vi "PH_Switch.set Default.vi"(0 "i ref in":refnum<vi>, 5 "error in":errorcluster) -> (14 "i ref out":refnum<vi>, 19 "error out":errorcluster)   [LabVIEW 2014, in "PH_Switch.lvlib"]
doc: "This VI sets the default value."
uses:
  PH_Switch.lvlib
  CS_Core/CSSystem/CSSystemLib/CSSystemLib.lvlib
  CS_Core/BaseProcess/BaseProcess.lvlib
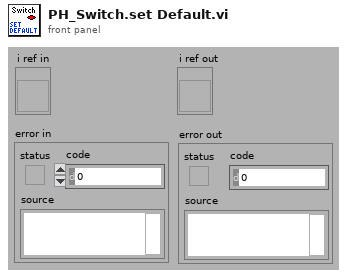
[diagram p1: front panel]
types:
  T1 = typedef "BaseProcess.lvlib/BaseProcess.i attribute.ctl" = cluster{"EventStatus":string, "EventError":i32, "PresetEvtWatchD":i32, "PresetPdcWatchD":i32, "EventTimeout":i32, "PeriodicInterval":i32, "Interface":string[], "Address":string[], "Special":string[], "PeriodicError":i32, "PeriodicStatus":string, "SuperProc":string, "Descriptors":T2[], "CaseRef":refnum<vi>, "PdcRef":refnum<vi>, "Thread Ref":refnum<vi>, "eventErrorID":i32, "eventStatusID":i32, "periodicErrorID":i32, "periodicStatusID":i32, "pdcCtrID":i32}
  T2 = typedef "BaseProcess.lvlib/BaseProcess.descriptor definition.ctl" = cluster{"selector":string, "descriptor":T3}
  T3 = typedef "BaseProcess.lvlib/BaseProcess.descriptor string definition.ctl" = string
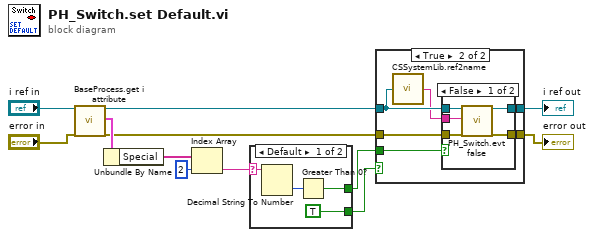
[diagram p0: block diagram]
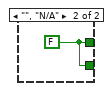
[diagram p2: hidden frame]
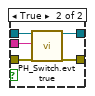
[diagram p4: hidden frame]
diagram:
  n1 = call "BaseProcess.get i attribute.vi"("i ref in"="i ref in", "error in (no error)"="error in") -> ("i ref out"=w2:refnum<vi>, "i attribute"=w10:T1, "error out"=w1:errorcluster)  [unwired: 15 in]
  n2 = Unbundle By Name(w10) -> ("Special"=w9:string[])
  n3 = Index Array(array=w9, index=2) -> (element=w7:string)
  n4 = case shown="Default" w7 {
    selector: w7 -> [w15 _]
    tunnel: [TRUE w17] -> w6
    tunnel: [w13 w17] -> w5
    frame Default {
      n5 = Decimal String To Number(string=w15) -> (number=w14:i32)  [unwired: 2 in, 1 out]
      n6 = Greater Than 0?(x=w14) -> (x > 0?=w13:bool)
    }
    frame "", "N/A" {
      w17 = FALSE
    }
  }
  n7 = case shown="True" w6 {
    tunnel: [w19 w25] -> w11
    tunnel: w1 -> [w18 w24]
    tunnel: [w18 w23] -> w12
    tunnel: w5 -> [_ w22]
    tunnel: w2 -> [w19 w21]
    frame False {
    }
    frame True {
      n8 = call "CSSystemLib.ref2name.vi"("obj refnum"=w21) -> ("name"=w20:string)
      n9 = case shown="False" w22 {
        tunnel: w21 -> [w30 w35]
        tunnel: [w29 w34] -> w25
        tunnel: w24 -> [w28 w33]
        tunnel: [w27 w32] -> w23
        tunnel: w20 -> [w26 w31]
        frame False {
          n10 = call "PH_Switch.evt false.vi"("i ref in"=w30, "Instance"=w26, "error in (no error)"=w28) -> ("i ref out"=w29:refnum<vi>, "error out"=w27:errorcluster)  [unwired: 15 in]
        }
        frame True {
          n11 = call "PH_Switch.evt true.vi"("i ref in"=w35, "Instance"=w31, "error in (no error)"=w33) -> ("i ref out"=w34:refnum<vi>, "error out"=w32:errorcluster)  [unwired: 15 in]
        }
      }
    }
  }
  "error out" <- w12
  "i ref out" <- w11
